vi "SetControlWord.vi"(8 "error in (no error)":errorcluster, 11 "Motor Base in":refnum<class "Motor Base.lvclass">) -> (0 "error out":errorcluster, 3 "Motor Base out":refnum<class "Motor Base.lvclass">)   [LabVIEW 2016, in "Motor Base.lvlib" / "Motor Base.lvclass"]
uses:
  Motor Base.lvclass
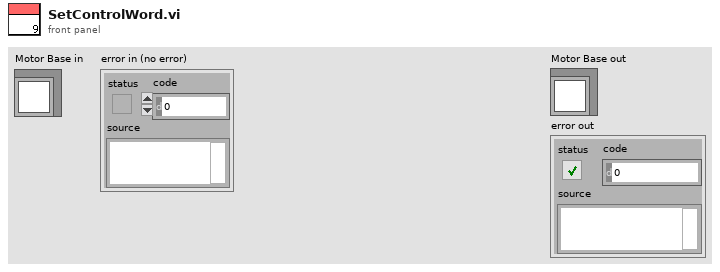
[diagram p1: front panel]
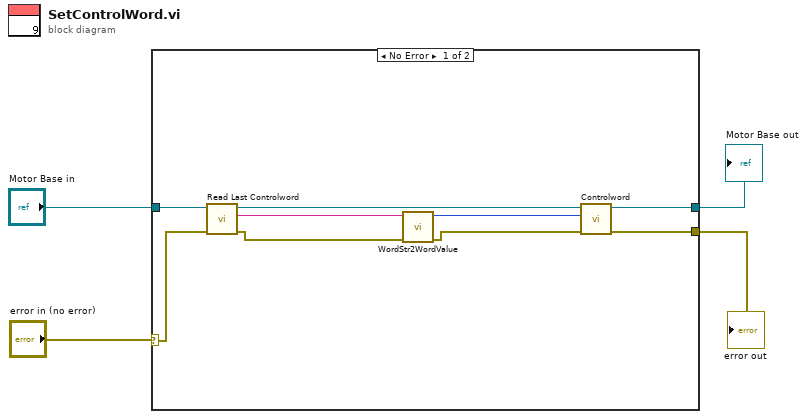
[diagram p0: block diagram]
diagram:
  n1 = case shown="No Error" "error in (no error)" {
    selector: "error in (no error)" -> [w5 w14]
    tunnel: "Motor Base in" -> [w11 w15]
    tunnel: [w7 w15] -> w3
    tunnel: [w6 w14] -> w2
    frame No Error {
      n2 = call-dynamic "Read Last Controlword.vi"("error in (no error)"=w5, "Motor Base in"=w11) -> ("error out"=w10:errorcluster, "Controlword"=w9:string, "Motor Base out"=w8:refnum<class "Motor Base.lvclass">)  [unwired: 7 in]
      n3 = call "WordStr2WordValue.vi"("error in (no error)"=w10, "Word"=w9) -> ("error out"=w12:errorcluster, "Word Value"=w13:i32)  [unwired: 8 in]
      n4 = call-dynamic "Controlword.vi"("error in"=w12, "Data"=w13, "Motor Base in"=w8) -> ("error out"=w6:errorcluster, "Motor Base out"=w7:refnum<class "Motor Base.lvclass">)  [unwired: 6 in, 1 out]
    }
    frame Error {
    }
  }
  "Motor Base out" <- w3
  "error out" <- w2
